vi "PlayerMain.vi"() -> ()   [LabVIEW 2010, in "Player.lvlib"]
uses:
  Player.lvlib
  CLIB/CThread/XNodes/referencenode/CThread VI Reference.xnode
  CLIB/CThread/XNodes/terminalnode/CThread VI Terminal Node.xnode
  CLIB/CThread/Base/CThread Base - VI Reference.vi
  CLIB/CThread/Base/CThread Base - Set Conditional Terminal.vi
  Components/Components.lvlib
  Timer Extensions/timerExts.lvlib
  CLIB/CThread/CThread.lvlib
panel:
  out "Timer":T1
  in  "CurrentTime":i16
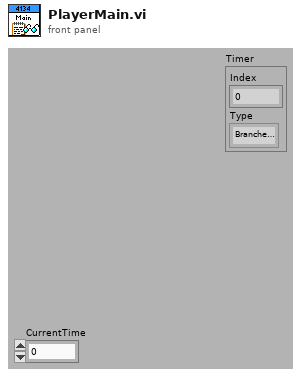
[diagram p1: front panel]
types:
  T1 = cluster{"Index":u16, "Type":enum8{"Branched Timer", "NXT Timer"}}
  T2 = typedef "NXT_FileStatusCodes.ctl" = u16
  T3 = typedef "LVHSConnector.ctl" = cluster{"Hardware":string, "Flattened String":string}
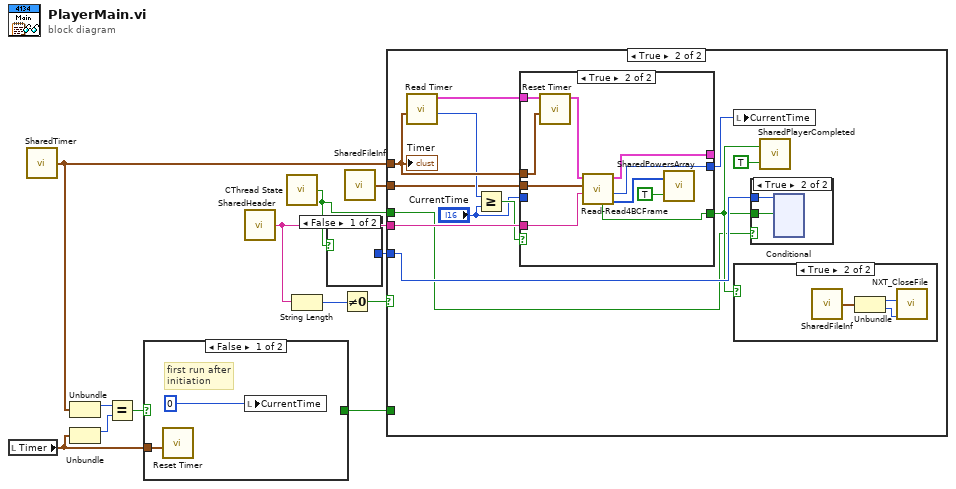
[diagram p0: block diagram]
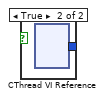
[diagram p2: hidden frame]
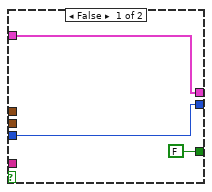
[diagram p7: hidden frame]
diagram:
  n1 = local read "Timer"() -> (w3:T1)
  n2 = call "SharedTimer.vi"() -> ("Timer"=w8:T1)  [unwired: 2 in]
  n3 = Unbundle(w8) -> ("Index"=w7:u16)  [unwired: 1 out]
  n4 = Unbundle(w3) -> ("Index"=w6:u16)  [unwired: 1 out]
  n5 = Equal?(x=w7, y=w6) -> (x = y?=w5:bool)
  n6 = case shown="False" w5 {
    selector: w5 -> [_ w15]
    tunnel: [_ w15] -> w4
    tunnel: w3 -> [w13 _]
    frame False {
      # "first run after\ninitiation"
      n7 = call "Reset Timer.vi"("Branched Timer Index"=w13) -> ()  [unwired: 10 in, 1 out]
      n8 = local write "CurrentTime"(i16 0 ("CurrentTime")) -> ()
    }
    frame True {
    }
  }
  n9 = call "SharedHeader.vi"() -> ("Header"=w2:string)  [unwired: 2 in]
  n10 = call "CThread State.vi"() -> ("Active?"=w1:bool)  [unwired: 4 in, 1 out]
  n11 = String Length(string=w2) -> (length=w11:i32)
  n12 = case shown="False" w1 {
    tunnel: [_ w16] -> w10
    frame False {
    }
    frame True {
      n13 = xnode "CThread VI Reference"() -> ("PlayerMain.vi"=w16:i32)
    }
  }
  n14 = Not Equal To 0?(x=w11) -> (x != 0?=w12:bool)
  n15 = call "SharedFileInf.vi"() -> ("FileInf"=w9:cluster{"Error in":T2, "File Handle in":u8})  [unwired: 2 in]
  n16 = case shown="True" w12 {
    tunnel: w2 -> [_ w31]
    tunnel: w8 -> [_ w30]
    tunnel: w10 -> [_ w23]
    tunnel: w9 -> [_ w22]
    tunnel: w4 -> [_ _]
    tunnel: w1 -> [_ w20]
    frame False {
    }
    frame True {
      n17 = call "Read Timer.vi"("Branched Timer Index"=w30) -> ("Value (msec)"=w24:u32, "NXT"=w25:T3)  [unwired: 9 in]
      n18 = Greater Or Equal?(x=w24, y="CurrentTime") -> (x >= y?=w29:bool)
      n19 = case shown="True" w29 {
        tunnel: w25 -> [w39 w47]
        tunnel: [w41 w51] -> w26
        tunnel: "CurrentTime" -> [w41 _]
        tunnel: [FALSE w50] -> w21
        tunnel: [w39 w45] -> _
        tunnel: w31 -> [_ w43]
        tunnel: w30 -> [_ w46]
        tunnel: w22 -> [_ w44]
        frame False {
        }
        frame True {
          n20 = call "Reset Timer.vi"("Branched Timer Index"=w46, "NXT"=w47) -> ("NXT"=w42:T3)  [unwired: 9 in]
          n21 = call "Read-Read4BCFrame.vi"("Header"=w43, "File Information"=w44, "NXT"=w42) -> ("Array"=w49:i16[], "Time"=w51:u32, "NXT"=w45:T3, "EOF?"=w50:bool)  [unwired: 4 in, 1 out]
          n22 = call "SharedPowersArray.vi"("Write?"=TRUE, "PowersInput"=w49) -> ()  [unwired: 1 out]
        }
      }
      n23 = local write "CurrentTime"(w26) -> ()
      n24 = case shown="True" w21 {
        frame False {
        }
        frame True {
          n25 = call "SharedFileInf.vi"() -> ("FileInf"=w38:cluster{"Error in":T2, "File Handle in":u8})  [unwired: 2 in]
          n26 = Unbundle(w38) -> ("Error in"=w37:T2, "File Handle in"=w36:u8)
          n27 = call <vilib>:"NXT_CloseFile.vi"("Error in"=w36, "File Handle"=w37) -> ()  [unwired: 8 in, 2 out]
        }
      }
      n28 = case shown="True" w20 {
        tunnel: w23 -> [_ w33]
        tunnel: w21 -> [_ w32]
        frame False {
        }
        frame True {
          n29 = xnode "Conditional"("CLIB VI Reference"=w33, "Stop?"=w32) -> ()  [unwired: 1 out]
        }
      }
      n30 = call "SharedPlayerCompleted.vi"("Write?"=TRUE, "PlayerCompletedInput"=w21) -> ()  [unwired: 1 out]
      "Timer" <- w30
    }
  }
